vi "rmad skredstorrelser initfile.vi"(0 "initfile":string="rmad config.ini", 11 "error in (no error)":errorcluster) -> (4 "Trafikkontroll terskelverdier":T1(array[cluster]), 6 "Stredstørrelser terskelverdier":T2(array[cluster]), 8 "num geofon noder":u32, 14 "ini file":path, 15 "error out":errorcluster)   [LabVIEW 2017]
uses:
  <vilib>/Utility/config.llb/Read Key (U32).vi
  <vilib>/Utility/config.llb/NI_LVConfig.lvlib
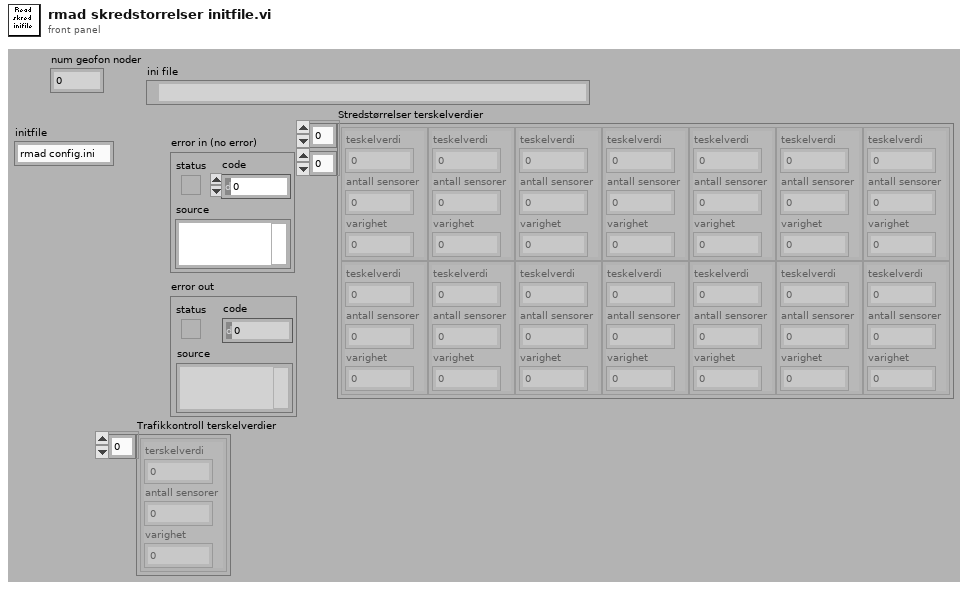
[diagram p1: front panel]
types:
  T1 = cluster{"terskelverdi":u32, "antall sensorer":u32, "varighet":u32}[]
  T2 = cluster{"teskelverdi":u32, "antall sensorer":u32, "varighet":u32}[][]
  T3 = typedef "NI_LVConfig.lvlib/Config Data RefNum.ctl" = refnum<k1>
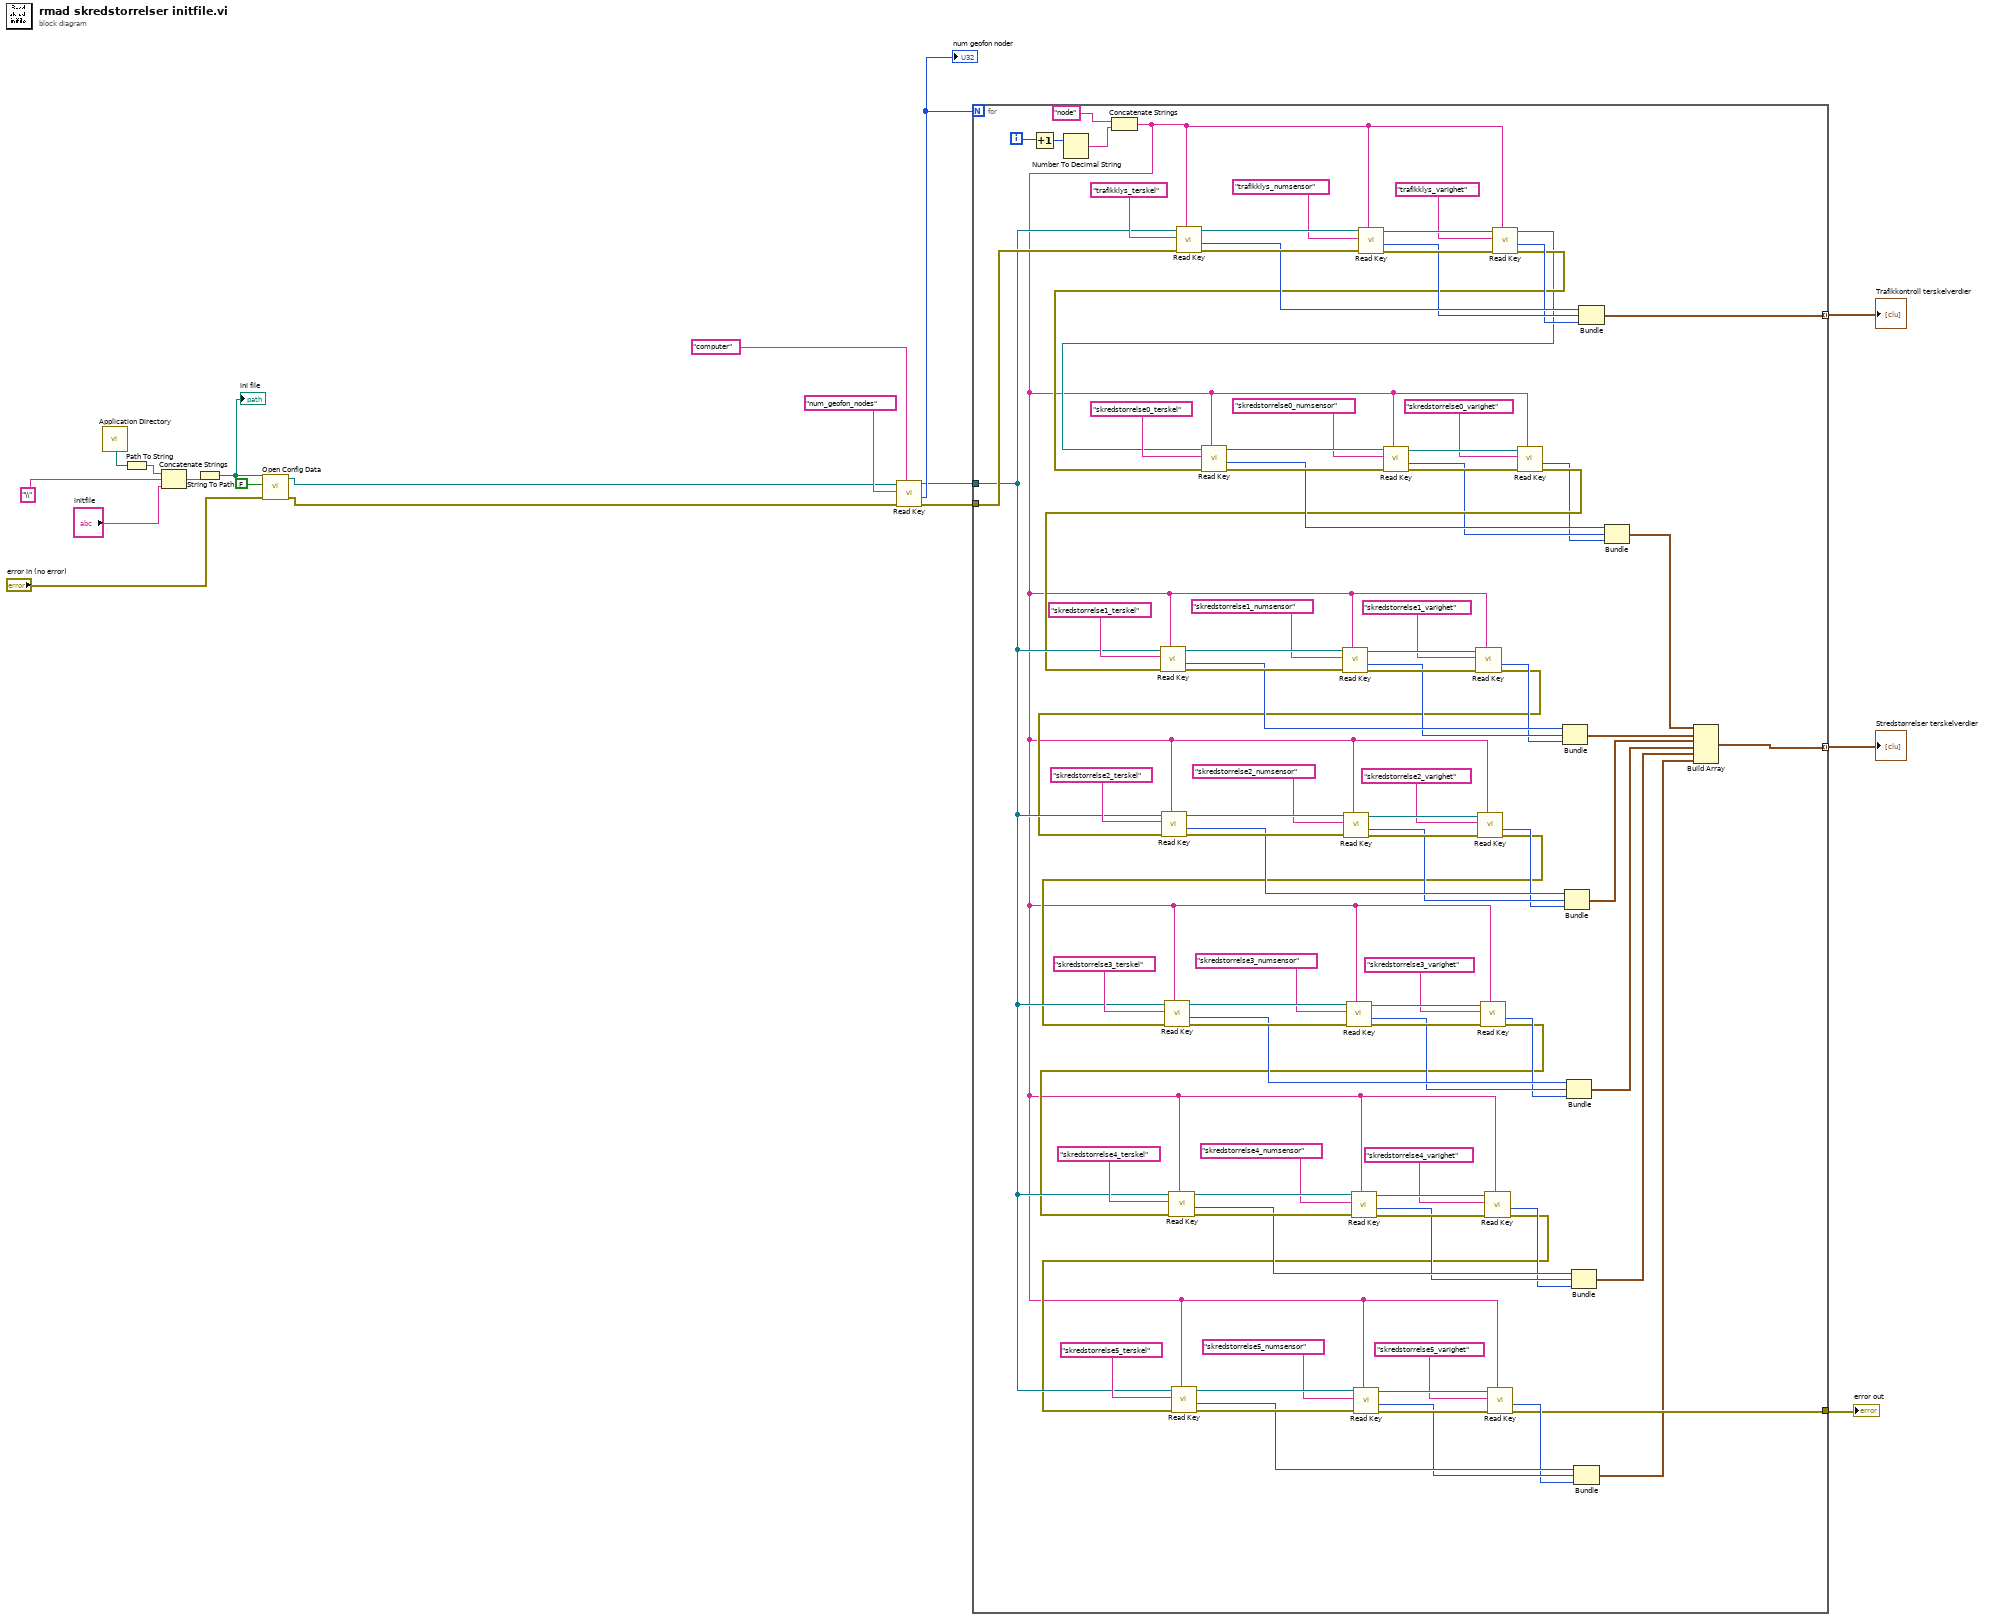
[diagram p0: block diagram]
diagram:
  n1 = call <vilib>:"Application Directory.vi"() -> ("Application Directory"=w18:path)
  n2 = Path To String(path=w18) -> (string=w17:string)
  n3 = Concatenate Strings(w17, "\\", "initfile") -> (w15:string)
  n4 = String To Path(string=w15) -> (path=w14:path)
  "ini file" <- w14
  n5 = call <vilib>:"Open Config Data.vi"("error in (no error)"="error in (no error)", "create file if necessary (T)"=FALSE, "configuration file path"=w14) -> ("error out"=w6:errorcluster, "refnum"=w5:T3)  [unwired: 6 in, 1 out]
  n6 = call-poly <vilib>:"Read Key.vi"("section"="computer", "error in (no error)"=w6, "key"="num_geofon_nodes", "refnum"=w5) -> ("error out"=w9:errorcluster, "value"=w10:u32, "refnum out"=w8:T3)  [unwired: 4 in, 1 out]
  "num geofon noder" <- w10
  n7 = for {
    N: w10 -> [_]
    tunnel: w9 -> [w106]
    tunnel: w8 -> [w46]
    tunnel: [w41] -> w4
    tunnel: [w40] -> w2 mode=indexing
    tunnel: [w34] -> w3 mode=indexing
    i -> [w108]
    n8 = Increment(x=w108) -> (x+1=w107:i32)
    n9 = Number To Decimal String(number=w107) -> (decimal integer string=w109:string)  [unwired: 1 in]
    n10 = Concatenate Strings("node" ("string"), w109) -> (w22:string)
    n11 = call-poly <vilib>:"Read Key.vi"("section"=w22, "error in (no error)"=w106, "key"="trafikklys_terskel" ("section"), "refnum"=w46) -> ("error out"=w105:errorcluster, "value"=w99:u32, "refnum out"=w104:T3)  [unwired: 4 in, 1 out]
    n12 = call-poly <vilib>:"Read Key.vi"("section"=w22, "error in (no error)"=w105, "key"="trafikklys_numsensor", "refnum"=w104) -> ("error out"=w103:errorcluster, "value"=w98:u32, "refnum out"=w102:T3)  [unwired: 4 in, 1 out]
    n13 = call-poly <vilib>:"Read Key.vi"("section"=w22, "error in (no error)"=w103, "key"="trafikklys_varighet", "refnum"=w102) -> ("error out"=w25:errorcluster, "value"=w97:u32, "refnum out"=w23:T3)  [unwired: 4 in, 1 out]
    n14 = call-poly <vilib>:"Read Key.vi"("section"=w22, "error in (no error)"=w25, "key"="skredstorrelse0_terskel" ("section"), "refnum"=w23) -> ("error out"=w32:errorcluster, "value"=w26:u32, "refnum out"=w31:T3)  [unwired: 4 in, 1 out]
    n15 = call-poly <vilib>:"Read Key.vi"("section"=w22, "error in (no error)"=w32, "key"="skredstorrelse0_numsensor", "refnum"=w31) -> ("error out"=w30:errorcluster, "value"=w21:u32, "refnum out"=w29:T3)  [unwired: 4 in, 1 out]
    n16 = call-poly <vilib>:"Read Key.vi"("section"=w22, "error in (no error)"=w30, "key"="skredstorrelse0_varighet", "refnum"=w29) -> ("error out"=w24:errorcluster, "value"=w20:u32)  [unwired: 4 in, 2 out]
    n17 = call-poly <vilib>:"Read Key.vi"("section"=w22, "error in (no error)"=w24, "key"="skredstorrelse1_terskel" ("section"), "refnum"=w46) -> ("error out"=w95:errorcluster, "value"=w89:u32, "refnum out"=w94:T3)  [unwired: 4 in, 1 out]
    n18 = call-poly <vilib>:"Read Key.vi"("section"=w22, "error in (no error)"=w95, "key"="skredstorrelse1_numsensor", "refnum"=w94) -> ("error out"=w93:errorcluster, "value"=w88:u32, "refnum out"=w92:T3)  [unwired: 4 in, 1 out]
    n19 = call-poly <vilib>:"Read Key.vi"("section"=w22, "error in (no error)"=w93, "key"="skredstorrelse1_varighet", "refnum"=w92) -> ("error out"=w45:errorcluster, "value"=w87:u32)  [unwired: 4 in, 2 out]
    n20 = call-poly <vilib>:"Read Key.vi"("section"=w22, "error in (no error)"=w45, "key"="skredstorrelse2_terskel" ("section"), "refnum"=w46) -> ("error out"=w85:errorcluster, "value"=w79:u32, "refnum out"=w84:T3)  [unwired: 4 in, 1 out]
    n21 = call-poly <vilib>:"Read Key.vi"("section"=w22, "error in (no error)"=w85, "key"="skredstorrelse2_numsensor", "refnum"=w84) -> ("error out"=w83:errorcluster, "value"=w78:u32, "refnum out"=w82:T3)  [unwired: 4 in, 1 out]
    n22 = call-poly <vilib>:"Read Key.vi"("section"=w22, "error in (no error)"=w83, "key"="skredstorrelse2_varighet", "refnum"=w82) -> ("error out"=w44:errorcluster, "value"=w77:u32)  [unwired: 4 in, 2 out]
    n23 = call-poly <vilib>:"Read Key.vi"("section"=w22, "error in (no error)"=w44, "key"="skredstorrelse3_terskel" ("section"), "refnum"=w46) -> ("error out"=w75:errorcluster, "value"=w69:u32, "refnum out"=w74:T3)  [unwired: 4 in, 1 out]
    n24 = call-poly <vilib>:"Read Key.vi"("section"=w22, "error in (no error)"=w75, "key"="skredstorrelse3_numsensor", "refnum"=w74) -> ("error out"=w73:errorcluster, "value"=w68:u32, "refnum out"=w72:T3)  [unwired: 4 in, 1 out]
    n25 = call-poly <vilib>:"Read Key.vi"("section"=w22, "error in (no error)"=w73, "key"="skredstorrelse3_varighet", "refnum"=w72) -> ("error out"=w43:errorcluster, "value"=w67:u32)  [unwired: 4 in, 2 out]
    n26 = call-poly <vilib>:"Read Key.vi"("section"=w22, "error in (no error)"=w43, "key"="skredstorrelse4_terskel" ("section"), "refnum"=w46) -> ("error out"=w65:errorcluster, "value"=w59:u32, "refnum out"=w64:T3)  [unwired: 4 in, 1 out]
    n27 = call-poly <vilib>:"Read Key.vi"("section"=w22, "error in (no error)"=w65, "key"="skredstorrelse4_numsensor", "refnum"=w64) -> ("error out"=w63:errorcluster, "value"=w58:u32, "refnum out"=w62:T3)  [unwired: 4 in, 1 out]
    n28 = call-poly <vilib>:"Read Key.vi"("section"=w22, "error in (no error)"=w63, "key"="skredstorrelse4_varighet", "refnum"=w62) -> ("error out"=w42:errorcluster, "value"=w57:u32)  [unwired: 4 in, 2 out]
    n29 = call-poly <vilib>:"Read Key.vi"("section"=w22, "error in (no error)"=w42, "key"="skredstorrelse5_terskel" ("section"), "refnum"=w46) -> ("error out"=w55:errorcluster, "value"=w49:u32, "refnum out"=w54:T3)  [unwired: 4 in, 1 out]
    n30 = call-poly <vilib>:"Read Key.vi"("section"=w22, "error in (no error)"=w55, "key"="skredstorrelse5_numsensor", "refnum"=w54) -> ("error out"=w53:errorcluster, "value"=w48:u32, "refnum out"=w52:T3)  [unwired: 4 in, 1 out]
    n31 = call-poly <vilib>:"Read Key.vi"("section"=w22, "error in (no error)"=w53, "key"="skredstorrelse5_varighet", "refnum"=w52) -> ("error out"=w41:errorcluster, "value"=w47:u32)  [unwired: 4 in, 2 out]
    n32 = Bundle("value"=w89, "value"=w88, "value"=w87) -> (w39:cluster{"value":u32, "value":u32, "value":u32})  [unwired: 1 in]
    n33 = Bundle("value"=w79, "value"=w78, "value"=w77) -> (w38:cluster{"value":u32, "value":u32, "value":u32})  [unwired: 1 in]
    n34 = Bundle("value"=w69, "value"=w68, "value"=w67) -> (w37:cluster{"value":u32, "value":u32, "value":u32})  [unwired: 1 in]
    n35 = Bundle("value"=w59, "value"=w58, "value"=w57) -> (w36:cluster{"value":u32, "value":u32, "value":u32})  [unwired: 1 in]
    n36 = Bundle("value"=w49, "value"=w48, "value"=w47) -> (w35:cluster{"value":u32, "value":u32, "value":u32})  [unwired: 1 in]
    n37 = Bundle("value"=w99, "value"=w98, "value"=w97) -> (w40:cluster{"value":u32, "value":u32, "value":u32})  [unwired: 1 in]
    n38 = Bundle("value"=w26, "value"=w21, "value"=w20) -> (w19:cluster{"value":u32, "value":u32, "value":u32})  [unwired: 1 in]
    n39 = Build Array(w19, w39, w38, w37, w36, w35) -> (w34:cluster{"value":u32, "value":u32, "value":u32}[])
  }
  "error out" <- w4
  "Stredstørrelser terskelverdier" <- w3
  "Trafikkontroll terskelverdier" <- w2
